vi "Enqueue.vi"(6 "abort (F)":bool, 7 "is last element (F)":bool, 8 "element in":T1, 9 "size (0)":i32, 10 "is valid (T)":bool=TRUE, 11 "PipeData in":refnum<class "StreamData.lvclass">) -> (0 "element out":T1, 1 "count":i32, 2 "wait":refnum<k4>, 3 "PipeData out":refnum<class "StreamData.lvclass">, 4 "aborted?":bool)   [LabVIEW 2017, in "Stream-t'WPI_EncoderType.ctl'.lvlib" / "StreamData.lvclass"]
uses:
  <extravilib>/ChannelInstances/Stream-t'WPI_EncoderType.ctl'/StreamData.lvclass
  <vilib>/Rock Robotics/WPI/Encoder/WPI_EncoderType.ctl
  <extravilib>/ChannelInstances/Stream-t'WPI_EncoderType.ctl'/StreamData.lvclass/StreamData.ctl
  <resource>/ChannelSupport/_ChannelSupport/PipeLogic/PipeLogic.lvclass/PipeLogic.ctl
  <resource>/ChannelSupport/_ChannelSupport/PipeLogic/PipeLogic.lvclass
  <resource>/ChannelSupport/_ChannelSupport/_ChannelSupport.lvlib
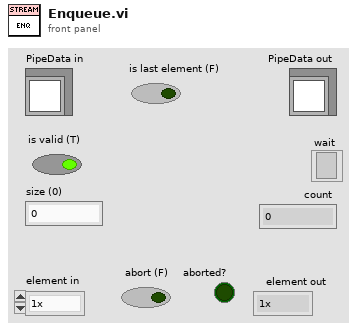
[diagram p1: front panel]
types:
  T1 = typedef "WPI_EncoderType.ctl" = enum16{"1x", "2x", "4x"}
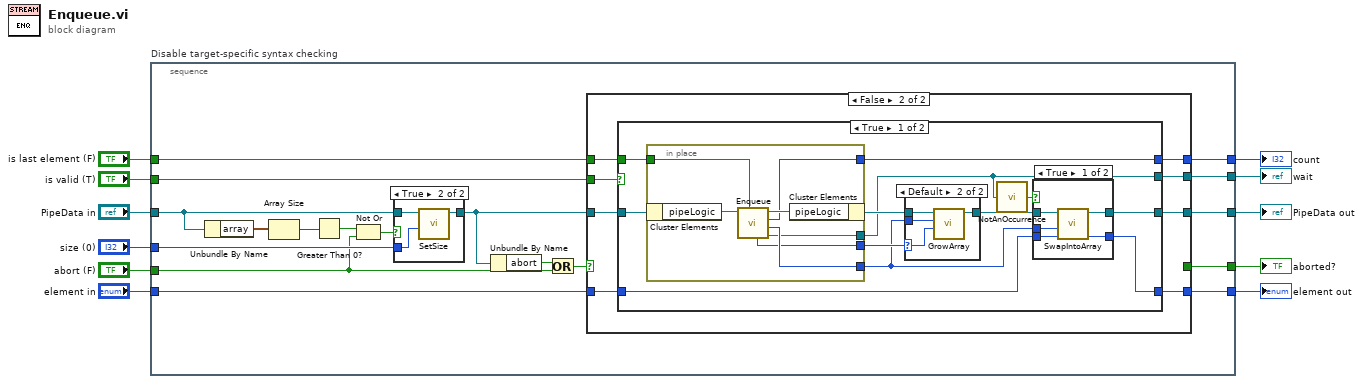
[diagram p0: block diagram]
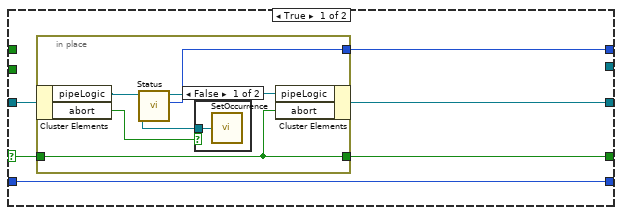
[diagram p3: hidden frame]
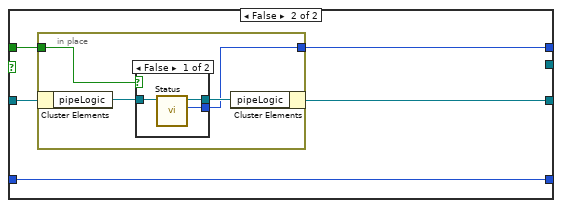
[diagram p7: hidden frame]
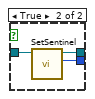
[diagram p8: hidden frame]
diagram:
  n1 = stacked-sequence "Disable target-specific syntax checking" {
    tunnel: [w29] -> w11
    tunnel: [w28] -> w10
    tunnel: [w27] -> w9
    tunnel: [w26] -> w8
    tunnel: [w25] -> w7
    tunnel: "is valid (T)" -> [w24]
    tunnel: "is last element (F)" -> [w23]
    tunnel: "element in" -> [w22]
    tunnel: "PipeData in" -> [w17]
    tunnel: "size (0)" -> [w16]
    tunnel: "abort (F)" -> [w14]
    frame #0 {
      n2 = Unbundle By Name(w17) -> ("array"=w21:cluster{"element":T1}[])
      n3 = Array Size(array=w21) -> (size(s)=w20:i32)
      n4 = Greater Than 0?(x=w20) -> (x > 0?=w19:bool)
      n5 = Not Or(1:w14, 2:w19) -> (0:w18:bool)
      n6 = case shown="True" w18 {
        tunnel: w17 -> [w30 w33]
        tunnel: [w30 w32] -> w15
        tunnel: w16 -> [_ w31]
        frame False {
        }
        frame True {
          n7 = call <resource>:"SetSize.vi"("size"=w31, "PipeData in"=w33) -> ("PipeData out"=w32:refnum<class "StreamData.lvclass">)  [unwired: 9 in]
        }
      }
      n8 = Unbundle By Name(w15) -> ("abort"=w13:bool)
      n9 = Or(x=w13, y=w14) -> (x .or. y?=w12:bool)
      n10 = case shown="False" w12 {
        selector: w12 -> [w35 _]
        tunnel: [w39 w54] -> w29
        tunnel: [w38 w53] -> w28
        tunnel: [w37 _] -> w27
        tunnel: [w34 w52] -> w26
        tunnel: [_ w51] -> w25
        tunnel: w24 -> [_ w50]
        tunnel: w23 -> [_ w49]
        tunnel: w22 -> [w34 w48]
        tunnel: w15 -> [w36 w47]
        frame True {
          n11 = in-place {
            in-place-border: [w43] -> w38
            in-place-border: [w40] -> w37
            in-place-border: w35 -> [w40]
            n12 = in-place-cluster #1(w36) -> ("pipeLogic"=w45:refnum<class "PipeLogic.lvclass">, "abort"=w42:bool)
            n13 = call <resource>:"Status.vi"("pipeLogic in"=w45) -> ("count"=w43:i32, "pipeLogic out"=w44:refnum<class "PipeLogic.lvclass">, "nonEmpty"=w41:refnum<k4>)  [unwired: 2 in, 6 out]
            n14 = case shown="False" w42 {
              tunnel: w41 -> [w46 _]
              frame False {
                n15 = call <resource>:"SetOccurrence.vi"("occurrence"=w46) -> ()  [unwired: 9 in]
              }
              frame True {
              }
            }
            n16 = in-place-cluster #1("pipeLogic"=w44, "abort"=w40) -> (w39:refnum<class "StreamData.lvclass">)
          }
        }
        frame False {
          n17 = case shown="True" w50 {
            tunnel: [w66 w90] -> w54
            tunnel: [w59 w89] -> w53
            tunnel: [w65 w86] -> w52
            tunnel: [w56 _] -> w51
            tunnel: w49 -> [w63 w88]
            tunnel: w48 -> [w57 w86]
            tunnel: w47 -> [w64 w87]
            frame True {
              n18 = in-place {
                in-place-border: w63 -> [w85]
                in-place-border: [w82] -> w59
                in-place-border: [w81] -> w58
                in-place-border: [w79] -> w60
                in-place-border: [w80] -> w56
                n19 = in-place-cluster #2(w64) -> ("pipeLogic"=w84:refnum<class "PipeLogic.lvclass">)
                n20 = call <resource>:"Enqueue.vi"("last element in"=w85, "pipeLogic in"=w84) -> ("wait"=w80:refnum<k4>, "index"=w81:i32, "count"=w82:i32, "pipeLogic out"=w83:refnum<class "PipeLogic.lvclass">, "grow"=w79:i32)  [unwired: 3 in, 2 out]
                n21 = in-place-cluster #2("pipeLogic"=w83) -> (w62:refnum<class "StreamData.lvclass">)
              }
              n22 = case shown="Default" w60 {
                selector: w60 -> [_ w75]
                tunnel: w62 -> [w74 w78]
                tunnel: [w74 w77] -> w61
                tunnel: w58 -> [_ w76]
                frame 0 {
                }
                frame Default {
                  n23 = call <extravilib>:"GrowArray.vi"("grow"=w75, "index"=w76, "PipeData in"=w78) -> ("PipeData out"=w77:refnum<class "StreamData.lvclass">)  [unwired: 8 in]
                }
              }
              n24 = call <resource>:"NotAnOccurrence.vi"("occurrence refnum"=w56) -> ("not an occurrence?"=w55:bool)
              n25 = case shown="True" w55 {
                tunnel: [w70 w72] -> w66
                tunnel: [w67 w73] -> w65
                tunnel: w57 -> [w69 w73]
                tunnel: w61 -> [w71 w72]
                tunnel: w58 -> [w68 _]
                frame True {
                  n26 = call <extravilib>:"SwapIntoArray.vi"("element in"=w69, "index"=w68, "PipeData in"=w71) -> ("element out"=w67:T1, "PipeData out"=w70:refnum<class "StreamData.lvclass">)  [unwired: 7 in]
                }
                frame False {
                  # "wait"
                }
              }
            }
            frame False {
              n27 = in-place {
                in-place-border: [w92] -> w89
                in-place-border: w88 -> [w91]
                n28 = in-place-cluster #3(w87) -> ("pipeLogic"=w94:refnum<class "PipeLogic.lvclass">)
                n29 = case shown="False" w91 {
                  tunnel: w94 -> [w97 w100]
                  tunnel: [w96 w99] -> w93
                  tunnel: [w95 w98] -> w92
                  frame False {
                    n30 = call <resource>:"Status.vi"("pipeLogic in"=w97) -> ("count"=w95:i32, "pipeLogic out"=w96:refnum<class "PipeLogic.lvclass">)  [unwired: 2 in, 7 out]
                  }
                  frame True {
                    n31 = call <resource>:"SetSentinel.vi"("pipeLogic in"=w100) -> ("count"=w98:i32, "pipeLogic out"=w99:refnum<class "PipeLogic.lvclass">)  [unwired: 9 in]
                  }
                }
                n32 = in-place-cluster #3("pipeLogic"=w93) -> (w90:refnum<class "StreamData.lvclass">)
              }
            }
          }
        }
      }
    }
  }
  "PipeData out" <- w11
  "aborted?" <- w9
  "count" <- w10
  "wait" <- w7
  "element out" <- w8
